vi "ReadEXCEL.vi"(8 "错误输入（无错误）":errorcluster, 9 "EXCEL 标签":string="Sheet1", 10 "路径":path) -> (0 "错误输出":errorcluster, 1 "数据":string[][](array[string]))   [LabVIEW 2018]
panel:
  in  "数组":string[][](array[string])
  in  "Excel._Worksheet":refnum<k7>
  in  "Excel._Application":refnum<k7>
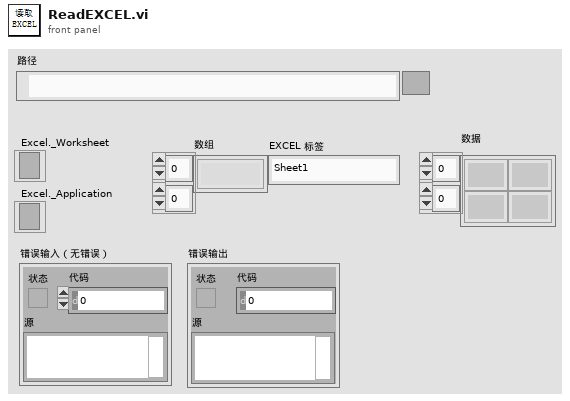
[diagram p1: front panel]
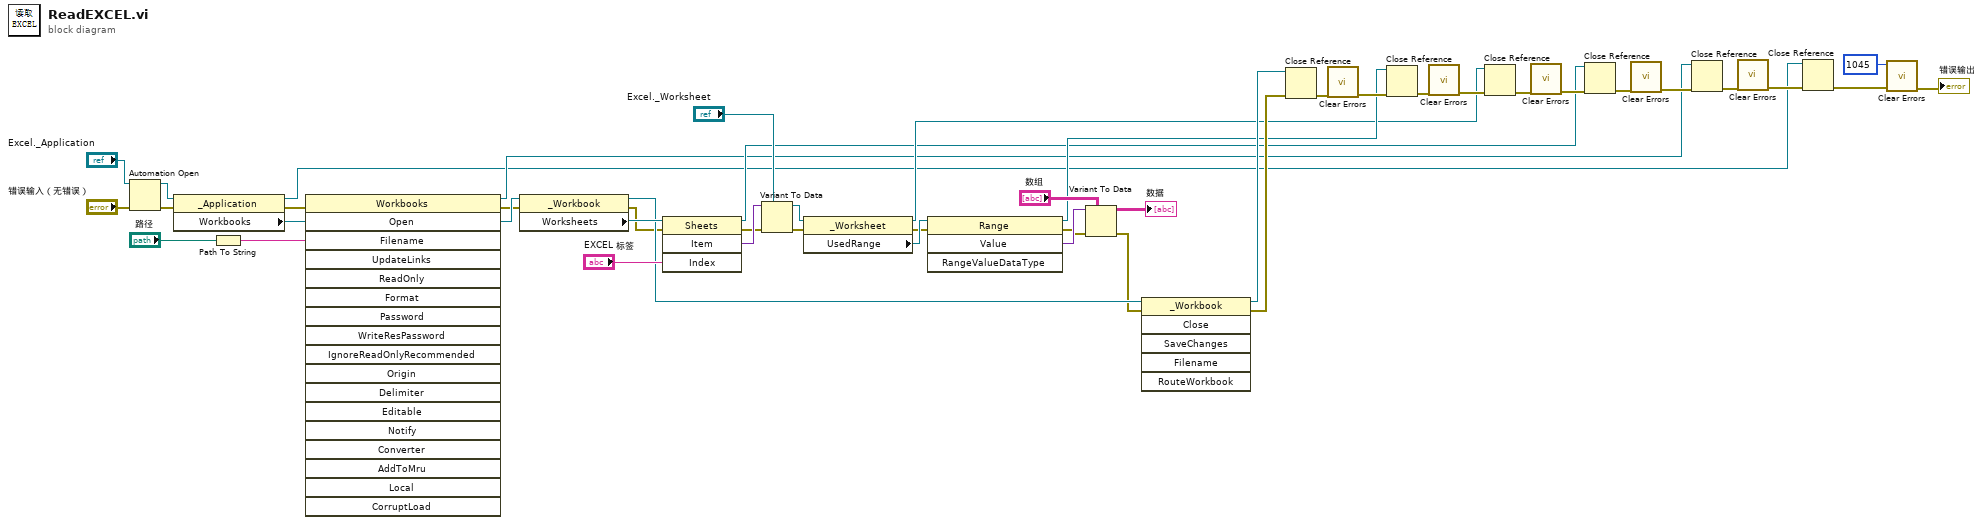
[diagram p0: block diagram]
diagram:
  n1 = Automation Open(error in (no error)="错误输入（无错误）", Automation Refnum="Excel._Application") -> (Automation Refnum=w5:refnum<k7>, error out=w46:errorcluster)  [unwired: 2 out]
  n2 = property class="_Application"(reference=w5, error in=w46) -> (reference out=w4:refnum<k7>, error out=w45:errorcluster, "Workbooks"=w28:refnum<k7>)
  n3 = Path To String(path="路径") -> (string=w27:string)
  n4 = invoke class="Workbooks" method="Open"(reference=w28, error in=w45, "Filename"=w27) -> (reference out=w7:refnum<k7>, error out=w43:errorcluster, "Open"=w44:refnum<k7>)  [unwired: 15 in, 15 out]
  n5 = property class="_Workbook"(reference=w44, error in=w43) -> (reference out=w26:refnum<k7>, error out=w22:errorcluster, "Worksheets"=w42:refnum<k7>)
  n6 = invoke class="Sheets" method="Item"(reference=w42, error in=w22, "Index"="EXCEL 标签") -> (reference out=w10:refnum<k7>, error out=w39:errorcluster, "Item"=w41:variant)  [unwired: 1 in, 1 out]
  n7 = Variant To Data(error in=w39, type="Excel._Worksheet", Variant=w41) -> (data=w38:refnum<k7>, error out=w35:errorcluster)
  n8 = property class="_Worksheet"(reference=w38, error in=w35) -> (reference out=w13:refnum<k7>, error out=w34:errorcluster, "UsedRange"=w37:refnum<k7>)
  n9 = invoke class="Range" method="Value"(reference=w37, error in=w34) -> (reference out=w14:refnum<k7>, error out=w33:errorcluster, "Value"=w36:variant)  [unwired: 2 in, 1 out]
  n10 = Variant To Data(error in=w33, type="数组", Variant=w36) -> (data=→"数据":string[][], error out=w25:errorcluster)
  n11 = invoke class="_Workbook" method="Close"(reference=w26, error in=w25) -> (reference out=w15:refnum<k7>, error out=w20:errorcluster)  [unwired: 4 in, 4 out]
  n12 = Close Reference(reference=w15, error in (no error)=w20) -> (error out=w21:errorcluster)
  n13 = call <vilib>:"Clear Errors.vi"("error in (no error)"=w21) -> ("error out"=w17:errorcluster)  [unwired: 5 in, 1 out]
  n14 = Close Reference(reference=w14, error in (no error)=w17) -> (error out=w19:errorcluster)
  n15 = call <vilib>:"Clear Errors.vi"("error in (no error)"=w19) -> ("error out"=w16:errorcluster)  [unwired: 5 in, 1 out]
  n16 = Close Reference(reference=w13, error in (no error)=w16) -> (error out=w18:errorcluster)
  n17 = call <vilib>:"Clear Errors.vi"("error in (no error)"=w18) -> ("error out"=w11:errorcluster)  [unwired: 5 in, 1 out]
  n18 = Close Reference(reference=w10, error in (no error)=w11) -> (error out=w12:errorcluster)
  n19 = call <vilib>:"Clear Errors.vi"("error in (no error)"=w12) -> ("error out"=w8:errorcluster)  [unwired: 5 in, 1 out]
  n20 = Close Reference(reference=w7, error in (no error)=w8) -> (error out=w9:errorcluster)
  n21 = call <vilib>:"Clear Errors.vi"("error in (no error)"=w9) -> ("error out"=w6:errorcluster)  [unwired: 5 in, 1 out]
  n22 = Close Reference(reference=w4, error in (no error)=w6) -> (error out=w3:errorcluster)
  n23 = call <vilib>:"Clear Errors.vi"("error in (no error)"=w3, "specific error code to clear (0: all)"=1045) -> ("error out"=→"错误输出":errorcluster)  [unwired: 4 in, 1 out]
